vi "sub_itertools-combinations.vi"(11 "N":i32) -> (3 "z_ids":cluster{"x":i32, "y":i32}[](array[cluster]))   [LabVIEW 2019]
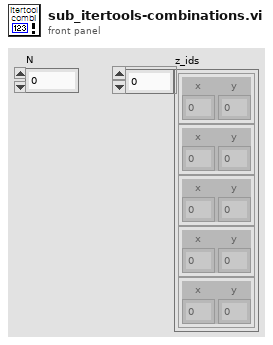
[diagram p1: front panel]
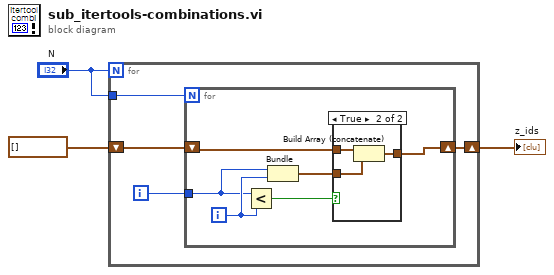
[diagram p0: block diagram]
diagram:
  n1 = for {
    N: "N" -> [_]
    shift-right: [w4] -> w1
    shift-left: cluster{"x":i32, "y":i32}[] [] -> [w6]
    tunnel: "N" -> [w7]
    i -> [w5]
    n2 = for {
      N: w7 -> [_]
      shift-right: [w8] -> w4
      shift-left: w6 -> [w9]
      tunnel: w5 -> [w12]
      i -> [w13]
      n3 = Less?(x=w12, y=w13) -> (x < y?=w11:bool)
      n4 = Bundle(w12, w13) -> (w10:cluster{i32, i32})  [unwired: 1 in]
      n5 = case shown="True" w11 {
        tunnel: w10 -> [_ w17]
        tunnel: w9 -> [w14 w16]
        tunnel: [w14 w15] -> w8
        frame False {
        }
        frame True {
          n6 = Build Array (concatenate)(w16, w17) -> (w15:cluster{"x":i32, "y":i32}[])
        }
      }
    }
  }
  "z_ids" <- w1
